vi "Global Log History Cacher.vi"(0 "Global Log Data":T3, 1 "Reset?":bool, 2 "Remove Immediately? (F)":bool, 3 "Time Format String":string="%<%H:%M:%S%3u>T", 5 "Length (10000)":i32=10000, 7 "With Periodic Info? (T)":bool=TRUE, 11 "Settings":T2={"threashold(#/s)"=1.9, "Check Peroid(s)"=1.0}, 12 "Level (Normal)":T1) -> (4 "String Cache":string)   [LabVIEW 2017, in "Communicable State Machine.lvlib"]
doc: "Saves the current input string to the cache. When the cached history strings exceed the maximum length limit, the oldest cached string will be overwritten. Use this VI for debugging CSM history states.\n\n-- <b>Controls</b> --\n- <b>Global Log Data</b>: Received global log information packet.\n- <b>Length (10000)</b>: Maximum string length for cached history strings.\n- <b>Level (Normal)</b>: Processing level. The default is <b>Normal</b>, which indicates standard processing. Higher levels omit different information to increase processing speed.\n- <b>Time Format String</b>: Timestamp format.\n- <b>With Periodic Info? (T)</b>: Whether to fold periodic logs.\n- <b>Remove Immediately? (F)</b>: Whether to immediately remove periodic folded information.\n- <b>Reset?</b>: Reset flag.\n- <b>Settings</b>: Periodic log configuration information. You can set detection period and periodic threshold to determine whether to fold.\n\n-- <b>Indicators</b> --\n- <b>String Cache</b>: Cached history strings."
uses:
  Communicable State Machine.lvlib
  _Support/Typedef/_CSM_GlobalLog_MSG.ctl
  _Support/Typedef/_CSM_Response Source Message.ctl
  _Support/Typedef/_CSM_GlobalLog_MSG_TYPE.ctl
  Periodic String Filter Setting.ctl
  _support/Periodic String Filter Level.ctl
  _Support/Common/Format Timestamp.vi
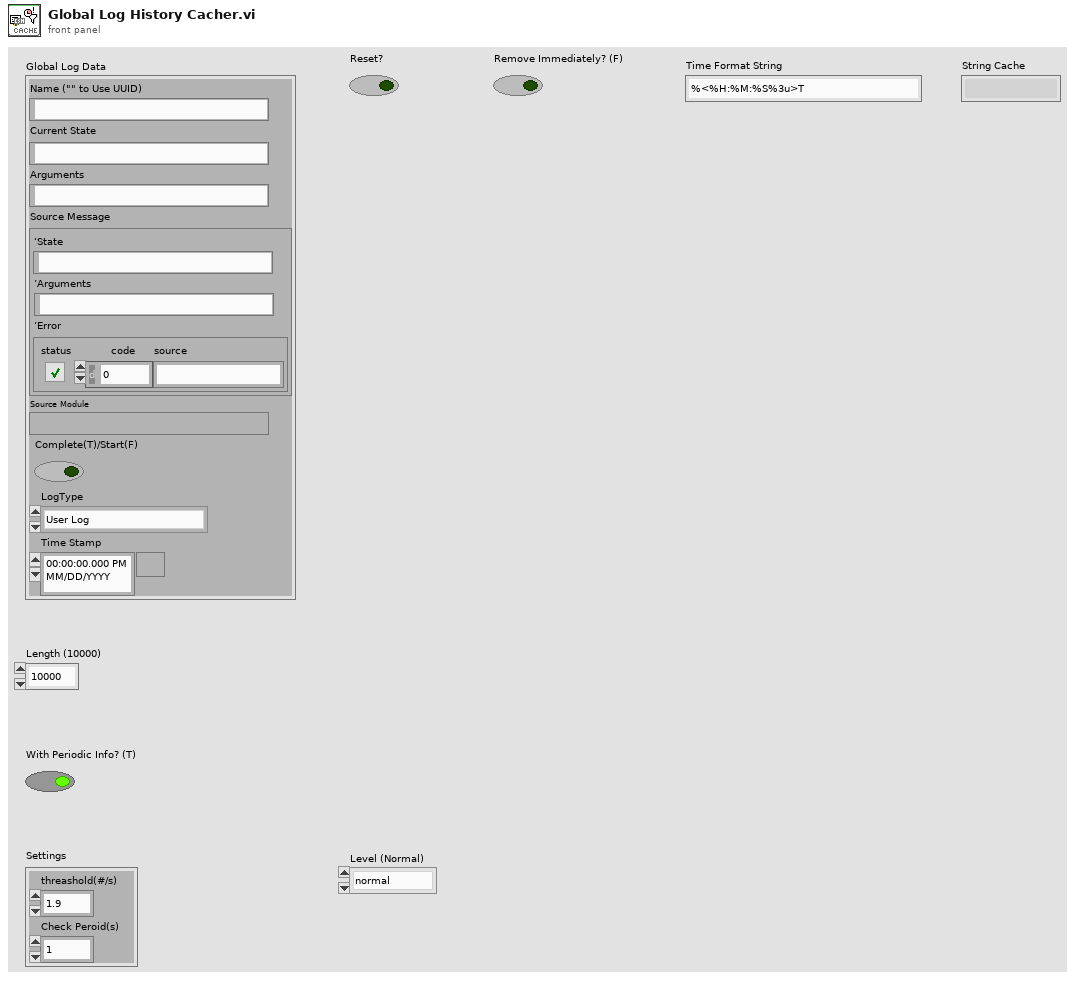
[diagram p1: front panel]
types:
  T1 = typedef "Communicable State Machine.lvlib/Periodic String Filter Level.ctl" = enum16{"normal", "L1", "L2", "L3", "L4"}
  T2 = typedef "Communicable State Machine.lvlib/Periodic String Filter Setting.ctl" = cluster{"threashold(#/s)":dbl, "Check Peroid(s)":dbl}
  T3 = typedef "Communicable State Machine.lvlib/_CSM_GlobalLog_MSG.ctl" = cluster{"Name (\"\" to Use UUID)":string, "Current State":string, "Arguments":string, "Source Message":T4, "Source Module":string, "Complete(T)/Start(F)":bool, "LogType":T5, "Time Stamp":timestamp}
  T4 = typedef "Communicable State Machine.lvlib/_CSM_Response Source Message.ctl" = cluster{"‘State":string, "’Arguments":string, "’Error":errorcluster}
  T5 = typedef "Communicable State Machine.lvlib/_CSM_GlobalLog_MSG_TYPE.ctl" = enum16{"User Log", "State Change", "Status", "Interrupt", "Register", "Unregister", "Error Log", "Module Created", "Module Destroyed", "Async Message", "No-Rep Async Message", "Sync Message"}
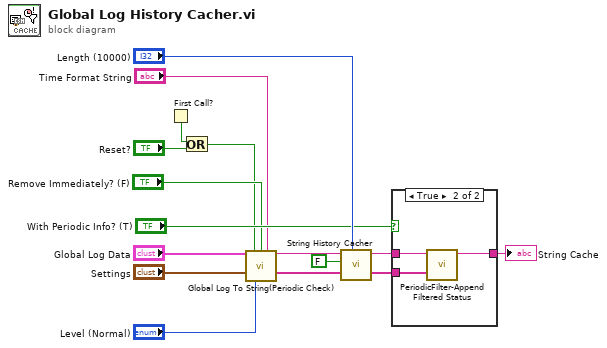
[diagram p0: block diagram]
diagram:
  n1 = First Call?() -> (First Call?: T/F=w10:bool)
  n2 = Or(x=w10, y="Reset?") -> (x .or. y?=w4:bool)
  n3 = call "Global Log To String(Periodic Check).vi"("Cross CSM Data"="Global Log Data", "Reset?"=w4, "Remove Immediately? (F)"="Remove Immediately? (F)", "Time Format String"="Time Format String", "Settings"="Settings", "Level (Normal)"="Level (Normal)") -> ("String"=w8:string, "Periodic Info"=w2:string[])  [unwired: 8 in]
  n4 = call "String History Cacher.vi"("Length"="Length (10000)", "Include Timestamp? (T)"=FALSE ("Include Timestamp(F)"), "String"=w8) -> ("String Cache"=w12:string)  [unwired: 8 in]
  n5 = case shown="True" "With Periodic Info? (T)" {
    tunnel: w12 -> [w16 w19]
    tunnel: [w16 w18] -> w11
    tunnel: w2 -> [_ w17]
    frame False {
    }
    frame True {
      n6 = call "PeriodicFilter-Append Filtered Status.vi"("Filtered Status"=w17, "String Cache In"=w19) -> ("String Cache Out"=w18:string)  [unwired: 9 in]
    }
  }
  "String Cache" <- w11
